vi "example_2_6_g.vi"() -> ()   [LabVIEW 2018]
panel:
  out "Array":bool[](array[boolean])
  in  "stop":bool
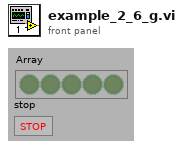
[diagram p1: front panel]
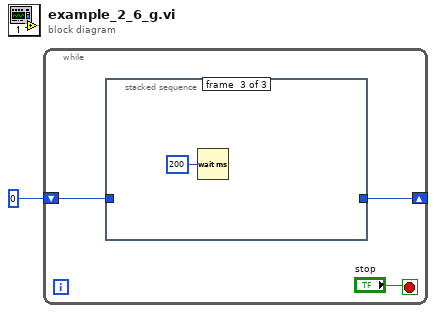
[diagram p0: block diagram]
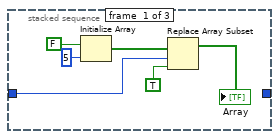
[diagram p2: hidden frame]
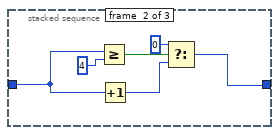
[diagram p3: hidden frame]
diagram:
  n1 = while {
    shift-right: [w2] -> _
    shift-left: 0 -> [w3]
    stop <- "stop" stop-if-true
    n2 = stacked-sequence {
      tunnel: w3 -> [w5 w12 _]
      tunnel: [_ w15 _] -> w2
      frame #0 {
        n3 = Initialize Array(FALSE, 5 ("Dimension Size")) -> (w8:bool[])
        n4 = Replace Array Subset(array=w8, new element=TRUE, index=w5) -> (→"Array":bool[])
      }
      frame #1 {
        n5 = Greater Or Equal?(x=w12, y=4) -> (x >= y?=w14:bool)
        n6 = Increment(x=w12) -> (x+1=w11:i32)
        n7 = Select(t=0, s=w14, f=w11) -> (s? t:f=w15:i32)
      }
      frame #2 {
        n8 = Wait (ms)(milliseconds to wait=u32 200) -> ()  [unwired: 1 out]
      }
    }
  }
